vi "reg.vi"() -> (0 "String":string)   [LabVIEW 2023]
doc: "This is a subVi used to save and edit a regular expresson for the next processing"
panel:
  in  "Regular Expresson":string
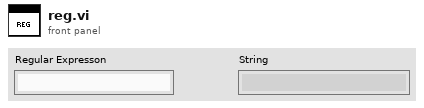
[diagram p1: front panel]
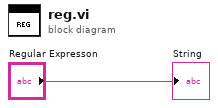
[diagram p0: block diagram]
diagram:
  "String" <- "Regular Expresson"
